vi "VI Server_Set Tab Ctr Page by Page Label.vi"(7 "TabCtr.Label":string="TESTs", 8 "error in":errorcluster, 9 "Page.Label":string, 11 "VI Server Cluster":T1={"VI Ref"=refnum, "Refs"=[], "Labels"=["Label", "Size", "Font", "Heght", "Width", "Ledding Denominator", "Ledding Nominator", "Label Number", "Microstep Resolution", "X", "Y", "Z", "Italic?", "Underlined?"]}) -> (0 "error out":errorcluster, 3 "VI Server Cluster.DUP":T1={"VI Ref"=refnum, "Refs"=[], "Labels"=["Label", "Size", "Font", "Heght", "Width", "Ledding Denominator", "Ledding Nominator", "Label Number", "Microstep Resolution", "X", "Y", "Z", "Italic?", "Underlined?"]})   [LabVIEW 2020, in "VI Server Toolkit LV2013.lvlib"]
doc: "Flips Tab Control page by the selected page name."
uses:
  VI Server Toolkit LV2013.lvlib
  VI Server Cluster.ctl
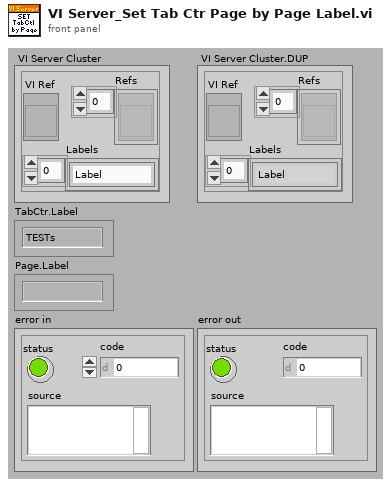
[diagram p1: front panel]
types:
  T1 = typedef "VI Server Toolkit LV2013.lvlib/VI Server Cluster.ctl" = cluster{"VI Ref":refnum<vi>, "Refs":refnum<vi>[], "Labels":string[]}
  T2 = enum32{"Page 1", "Page 2", "Page 3", "Page 4", "Page 5", "Page 6", "Page 7", "Page 8", "Page 9", "Page 10", "Page 11", "Page 12", "Page 13", "Page 14", "Page 15", "Page 16", "Page 17", "Page 18", "Page 19", "Page 20"}
  T3 = typedef "VI Server_RefsCluster.ctl" = cluster{"Labels":string[], "Refs":refnum<vi>[], "VI Ref":refnum<vi>}
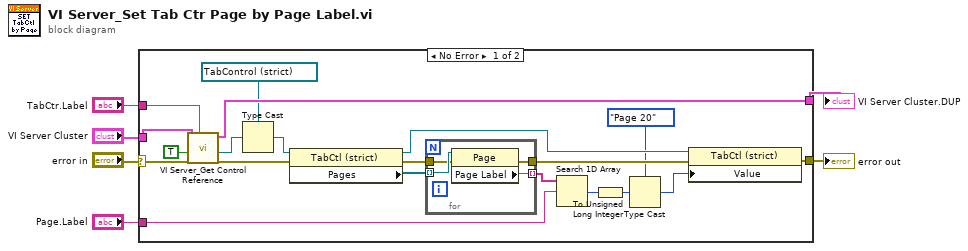
[diagram p0: block diagram]
diagram:
  n1 = case shown="No Error" "error in" {
    selector: "error in" -> [w12 w31]
    tunnel: [w26 w31] -> w6
    tunnel: "Page.Label" -> [w20 _]
    tunnel: "TabCtr.Label" -> [w18 _]
    tunnel: "VI Server Cluster" -> [w13 _]
    tunnel: [w11 _] -> w1
    frame No Error {
      n2 = call "VI Server_Get Control Reference.vi"("Label"=w18, "error in"=w12, "Single Instance (T)"=TRUE, "VI Server Cluster"=w13) -> ("error out"=w15:errorcluster, "Control Reference (Generic)"=w10:refnum<vi>, "VI Server Cluster.DUP"=w11:T3)  [unwired: 4 in, 1 out]
      n3 = Type Cast(type=refnum<vi> refnum ("Tab Control"), x=w10) -> (*(type *) &x=w14:refnum<vi>)
      n4 = property class="TabCtl (strict)"(reference=w14, error in=w15) -> (reference out=w22:refnum<vi>, error out=w17:errorcluster, "Pages"=w16:refnum<vi>[])
      n5 = for {
        tunnel: w16 -> [w30] mode=indexing
        tunnel: w17 -> [w29]
        tunnel: [w28] -> w21
        tunnel: [w27] -> w19 mode=indexing
        n6 = property class="Page"(reference=w30, error in=w29) -> (error out=w28:errorcluster, "Page Label"=w27:string)  [unwired: 1 out]
      }
      n7 = Search 1D Array(1D array=w19, element=w20) -> (index of element=w23:i32)  [unwired: 1 out]
      n8 = To Unsigned Long Integer(number=w23) -> (unsigned 32bit integer=w24:u32)
      n9 = Type Cast(type=T2."Page 20" ("Tab Control"), x=w24) -> (*(type *) &x=w25:T2)
      n10 = property class="TabCtl (strict)"(reference=w22, error in=w21, "Value"=w25) -> (error out=w26:errorcluster)  [unwired: 1 out]
    }
    frame Error {
    }
  }
  "error out" <- w6
  "VI Server Cluster.DUP" <- w1
